vi "Center Spin FL.vi"(0 "Wanted Angle":dbl, 1 "Current Angle":dbl) -> (7 "Motor Output":dbl format="%#_13g")   [LabVIEW 2020]
uses:
  <vilib>/addons/control/pid/pid.llb/PID (DBL).vi
  <vilib>/addons/control/pid/NI_PID_pid.lvlib
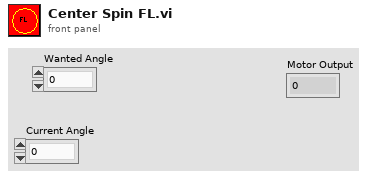
[diagram p1: front panel]
types:
  T1 = cluster{"proportional gain (Kc)":dbl, "integral time (Ti, min)":dbl, "derivative time (Td, min)":dbl}
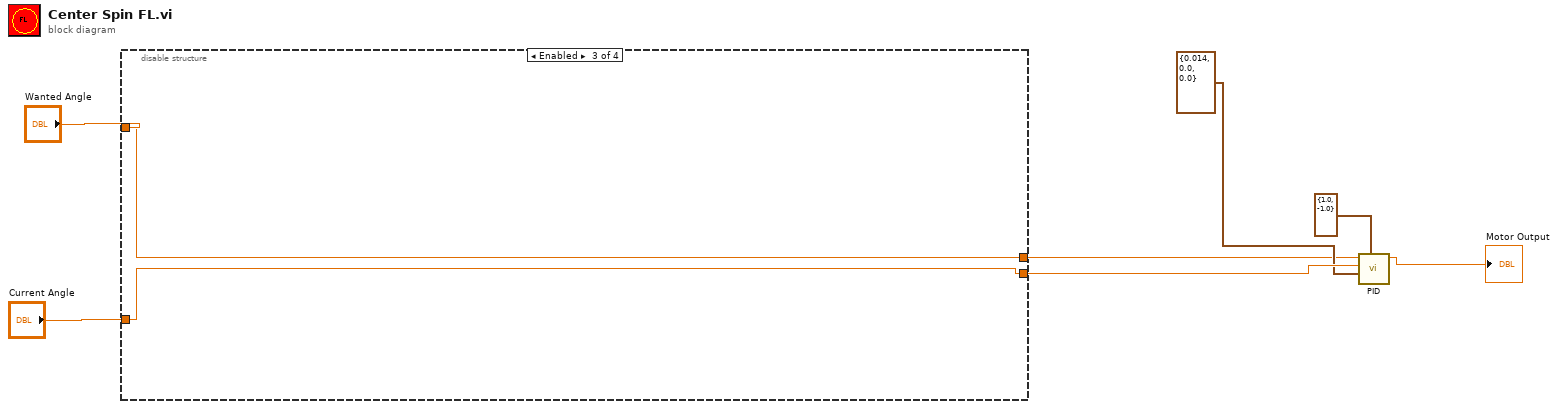
[diagram p0: block diagram]
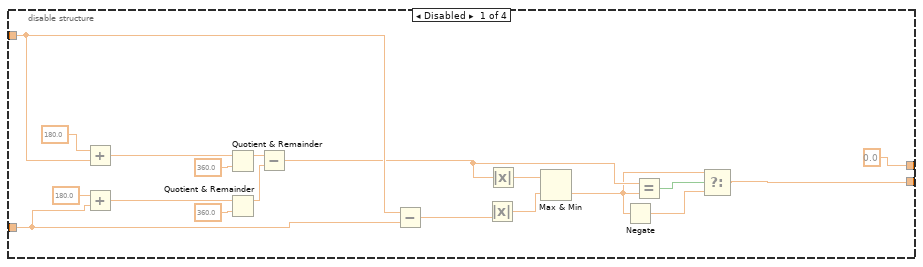
[diagram p2: hidden frame]
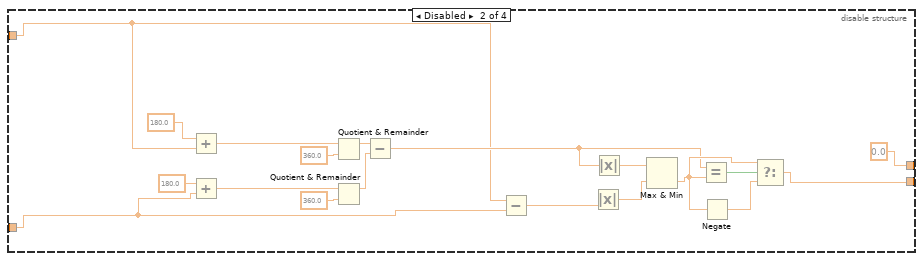
[diagram p3: hidden frame]
diagram:
  n1 = disable-structure shown="Enabled" {
    disable-tunnel: "Current Angle" -> [w26 w29 w46 w48]
    disable-tunnel: "Wanted Angle" -> [w25 w30 w47 w49]
    disable-tunnel: [w24 w27 w46 w48] -> w4
    disable-tunnel: [0.0 0.0 w47 w49] -> w1
    frame Disabled {
      n2 = Add(x=180.0, y=w25) -> (x+y=w10:dbl)
      n3 = Add(x=180.0, y=w26) -> (x+y=w11:dbl)
      n4 = Quotient & Remainder(x=w10, y=360.0) -> (x-y*floor(x/y)=w17:dbl)  [unwired: 1 out]
      n5 = Quotient & Remainder(x=w11, y=360.0) -> (x-y*floor(x/y)=w16:dbl)  [unwired: 1 out]
      n6 = Subtract(x=w17, y=w16) -> (x-y=w15:dbl)
      n7 = Subtract(x=w25, y=w26) -> (x-y=w18:dbl)
      n8 = Absolute Value(x=w18) -> (abs(x)=w12:dbl)
      n9 = Absolute Value(x=w15) -> (abs(x)=w9:dbl)
      n10 = Max & Min(x=w9, y=w12) -> (min(x,y)=w13:dbl)  [unwired: 1 out]
      n11 = Negate(x=w13) -> (-x=w14:dbl)
      n12 = Equal?(x=w15, y=w13) -> (x = y?=w23:bool)
      n13 = Select(t=w13, s=w23, f=w14) -> (s? t:f=w24:dbl)
    }
    frame Disabled {
      n14 = Add(x=180.0, y=w30) -> (x+y=w38:dbl)
      n15 = Add(x=180.0, y=w29) -> (x+y=w39:dbl)
      n16 = Quotient & Remainder(x=w38, y=360.0) -> (x-y*floor(x/y)=w41:dbl)  [unwired: 1 out]
      n17 = Quotient & Remainder(x=w39, y=360.0) -> (x-y*floor(x/y)=w40:dbl)  [unwired: 1 out]
      n18 = Subtract(x=w41, y=w40) -> (x-y=w31:dbl)
      n19 = Subtract(x=w30, y=w29) -> (x-y=w34:dbl)
      n20 = Absolute Value(x=w34) -> (abs(x)=w37:dbl)
      n21 = Absolute Value(x=w31) -> (abs(x)=w35:dbl)
      n22 = Max & Min(x=w35, y=w37) -> (min(x,y)=w33:dbl)  [unwired: 1 out]
      n23 = Equal?(x=w31, y=w33) -> (x = y?=w36:bool)
      n24 = Negate(x=w33) -> (-x=w32:dbl)
      n25 = Select(t=w33, s=w36, f=w32) -> (s? t:f=w27:dbl)
    }
    frame Enabled {
    }
    frame Disabled {
    }
  }
  n26 = call-poly <vilib>:"PID.vi"("output range"=cluster{"output high":dbl, "output low":dbl} {"output high"=1.0, "output low"=-1.0}, "PID gains"=T1 {"proportional gain (Kc)"=0.014, "integral time (Ti, min)"=0.0, "derivative time (Td, min)"=0.0} ("FR Pivot Motor PID gains"), "process variable"=w4, "setpoint"=w1) -> ("output"=→"Motor Output":dbl)  [unwired: 6 in, 1 out]
